vi "FTW-CodeGen-FindGObjects.vi"(0 "GObject to Traverse":refnum<vi>, 5 "Class Type Reference":variant, 7 "Maximum Expected Object Count":i32=64, 11 "error in":errorcluster) -> (6 "GObject Instances":refnum<vi>[](array[refnum]), 15 "error out":errorcluster)   [LabVIEW 2015]
panel:
  # "Inputs"
  # "Outputs"
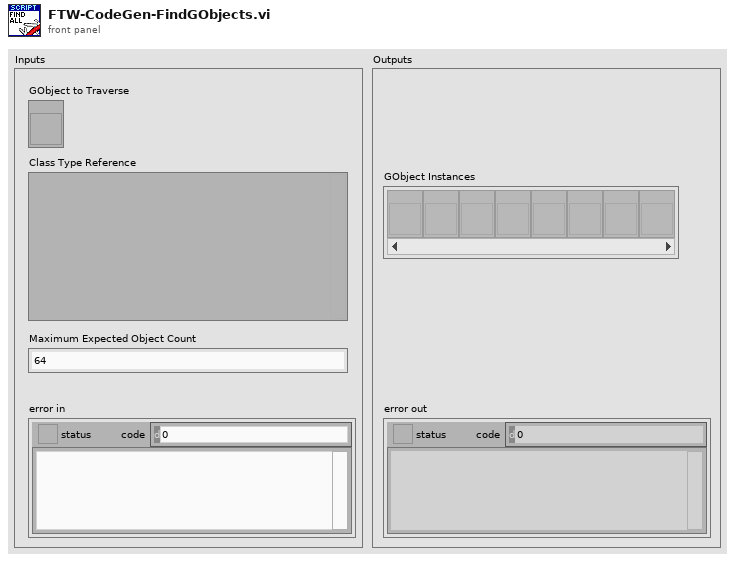
[diagram p1: front panel]
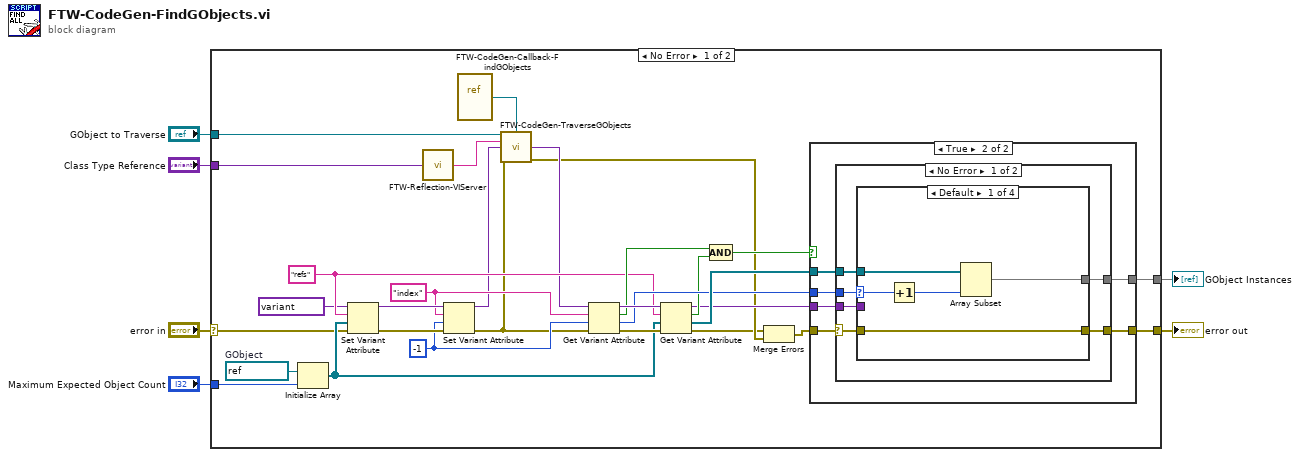
[diagram p0: block diagram]
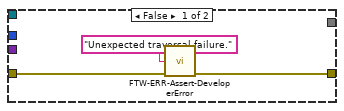
[diagram p2: hidden frame]
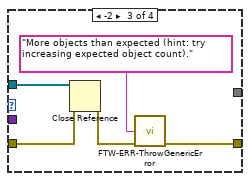
[diagram p4: hidden frame]
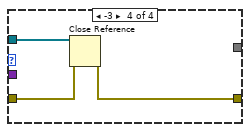
[diagram p5: hidden frame]
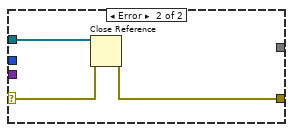
[diagram p6: hidden frame]
diagram:
  n1 = case shown="No Error" "error in" {
    selector: "error in" -> [w11 w69]
    tunnel: "GObject to Traverse" -> [w15 _]
    tunnel: [w36 _] -> w5
    tunnel: [w34 w69] -> w4
    tunnel: "Class Type Reference" -> [w33 _]
    tunnel: "Maximum Expected Object Count" -> [w35 _]
    frame No Error {
      w17 = refnum<vi> refnum  # GObject
      w20 = "refs" ("name")
      w26 = -1
      w19 = "index" ("name")
      n2 = Initialize Array(w17, w35) -> (w22:refnum<vi>[])
      n3 = Set Variant Attribute(Variant=variant, name=w20, value=w22, error in=w11) -> (Variant out=w31:variant, error out=w32:errorcluster)  [unwired: 1 out]
      n4 = call "FTW-Reflection-VIServer.vi"("VI Server Reference"=w33) -> ("Class Name"=w12:string)  [unwired: 11 in, 3 out]
      n5 = Set Variant Attribute(Variant=w31, name=w19, value=w26, error in=w32) -> (Variant out=w14:variant, error out=w10:errorcluster)  [unwired: 1 out]
      n6 = vi-ref "FTW-CodeGen-Callback-FindGObjects.vi"() -> (w16:refnum<vi>)
      n7 = call "FTW-CodeGen-TraverseGObjects.vi"("GObject to Traverse"=w15, "GObject Filter Callback"=w16, "Class Name"=w12, "Initial Context"=w14, "error in"=w10) -> ("Final Context"=w13:variant, "error out"=w9:errorcluster)  [unwired: 9 in]
      n8 = Get Variant Attribute(Variant=w13, name=w19, default value (empty Variant)=w26, error in=w10) -> (duplicate Variant=w30:variant, found=w23:bool, value=w25:i32, error out=w29:errorcluster)
      n9 = Get Variant Attribute(Variant=w30, name=w20, default value (empty Variant)=w22, error in=w29) -> (duplicate Variant=w21:variant, found=w24:bool, value=w27:refnum<vi>[], error out=w8:errorcluster)
      n10 = Compound Arithmetic op=AND(w23, w24) -> (w28:bool)
      n11 = Merge Errors(w8, w9) -> (w7:errorcluster)
      n12 = case shown="True" w28 {
        tunnel: [_ w45] -> w36
        tunnel: [w38 w44] -> w34
        tunnel: w7 -> [w39 w43]
        tunnel: w27 -> [_ w42]
        tunnel: w25 -> [_ w41]
        tunnel: w21 -> [_ w40]
        frame False {
          n13 = call "FTW-ERR-Assert-DeveloperError.vi"("Reason this error should never happen"="Unexpected traversal failure.", "error in"=w39) -> ("error out"=w38:errorcluster)  [unwired: 13 in]
        }
        frame True {
          n14 = case shown="No Error" w43 {
            selector: w43 -> [w47 w68]
            tunnel: w42 -> [w51 w66]
            tunnel: [w48 w67] -> w44
            tunnel: [w50 _] -> w45
            tunnel: w41 -> [w49 _]
            tunnel: w40 -> [w46 _]
            frame No Error {
              n15 = case shown="Default" w49 {
                selector: w49 -> [w54 _ _ _]
                tunnel: w51 -> [w56 _ w62 w65]
                tunnel: [w55 _ _ _] -> w50
                tunnel: [w53 w57 w59 w63] -> w48
                tunnel: w47 -> [w53 w57 w61 w64]
                tunnel: w46 -> [_ _ _ _]
                frame Default {
                  n16 = Increment(x=w54) -> (x+1=w52:i32)
                  n17 = Array Subset(array=w56, length=w52) -> (w55:refnum<vi>[])  [unwired: 1 in]
                }
                frame -1 {
                  # "No matching refs"
                }
                frame -2 {
                  n18 = Close Reference(reference=w62, error in (no error)=w61) -> (error out=w60:errorcluster)
                  n19 = call "FTW-ERR-ThrowGenericError.vi"("Error Message"="More objects than expected (hint: try increasing expected object count).", "error in"=w60) -> ("error out"=w59:errorcluster)  [unwired: 13 in]
                }
                frame -3 {
                  n20 = Close Reference(reference=w65, error in (no error)=w64) -> (error out=w63:errorcluster)
                }
              }
            }
            frame Error {
              n21 = Close Reference(reference=w66, error in (no error)=w68) -> (error out=w67:errorcluster)
            }
          }
        }
      }
    }
    frame Error {
    }
  }
  "error out" <- w4
  "GObject Instances" <- w5
